vi "Write Double.vi"(8 "error in (no error)":errorcluster, 9 "Numeric":dbl, 10 "Key":string="myhome/kitchen/temp", 11 "Zenoh in":refnum<class "Zenoh.lvclass">) -> (0 "error out":errorcluster)   [LabVIEW 2021, in "Zenoh.lvclass"]
doc: "Flatten a double and write to zenoh with provided key."
uses:
  Zenoh.lvclass
  Zenoh.lvclass/Zenoh.ctl
  58400e5e-2cc1-4aca-8f0f-3a78c0a2476e.vi
  SubVIs/Get Zenoh Path.vi
  58400e5e-2cc1-4aca-8f0f-3a78c0a2476e.vi/c28b0ead-42ad-4072-80a2-aca7f2bd7ce3.vi
  58400e5e-2cc1-4aca-8f0f-3a78c0a2476e.vi/d83f0d1e-b5f2-409c-a855-55c666a7c55e.vi
  58400e5e-2cc1-4aca-8f0f-3a78c0a2476e.vi/e02991d1-a06a-4e5e-a573-6dce97b92612.vi
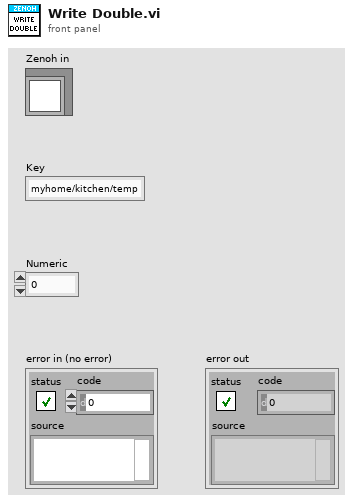
[diagram p1: front panel]
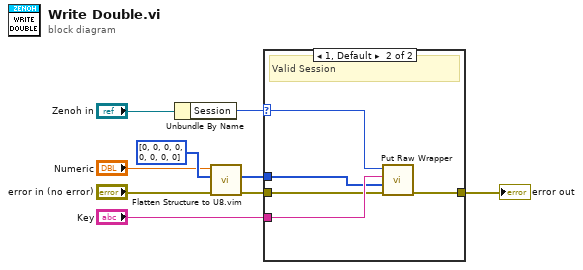
[diagram p0: block diagram]
diagram:
  n1 = Unbundle By Name("Zenoh in") -> ("Session"=w7:u64)
  n2 = call "Flatten Structure to U8.vim"("error in"="error in (no error)", "Flattened Data in"=u8[] [0, 0, 0, 0, 0, 0, 0, 0], "Data to Flatten in"="Numeric") -> ("error out"=w2:errorcluster, "Flattened Data out"=w5:u8[])  [unwired: 6 in, 1 out]
  n3 = case shown="1, Default" w7 {
    selector: w7 -> [_ w15]
    tunnel: "Key" -> [_ w14]
    tunnel: w2 -> [w10 w13]
    tunnel: [w10 w11] -> w6
    tunnel: w5 -> [_ w12]
    frame 0 {
      # "Invalid session"
    }
    frame 1, Default {
      # "Valid Session"
      n4 = call "Put Raw Wrapper.vi"("error in (no error)"=w13, "Raw Data"=w12, "key"=w14, "Session in"=w15) -> ("error out"=w11:errorcluster)  [unwired: 7 in]
    }
  }
  "error out" <- w6
